vi "Write INI.vi"   [LabVIEW 2025, in "Scripting Server.lvlib"]
uses:
  Scripting Server.lvlib
  <vilib>/Utility/config.llb/NI_LVConfig.lvlib
  <vilib>/Utility/config.llb/Write Key (Boolean).vi
types:
  T1 = typedef "NI_LVConfig.lvlib/Config Data RefNum.ctl" = refnum<k1>
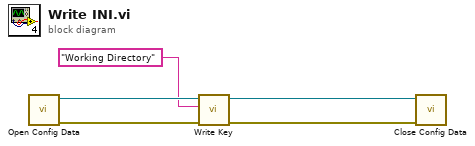
[diagram p0: block diagram]
diagram:
  n1 = call <vilib>:"Open Config Data.vi"() -> ("error out"=w4:errorcluster, "refnum"=w5:T1)  [unwired: 9 in, 1 out]
  n2 = call-poly <vilib>:"Write Key.vi"("error in (no error)"=w4, "key"="Working Directory", "refnum"=w5) -> ("error out"=w2:errorcluster, "refnum out"=w3:T1)  [unwired: 6 in, 1 out]
  n3 = call <vilib>:"Close Config Data.vi"("error in (no error)"=w2, "refnum"=w3) -> ()  [unwired: 8 in, 2 out]
